vi "WAV.vi"(0 "System no.":i32=1 min=1 max=4 step=1, 2 "Waveform":u16(ring) items=["SIN", "POL", "TAN", "PNT", "SIN_P", "LIN", "RAMP", "NOISE", "SWEEP"], 3 "Affected axes":string[](array[string]), 4 "Append? (&)":bool, 5 "Add? (+)":bool, 6 "No.of digits":i16=3, 7 "error in":errorcluster, 8 "Xo":i32, 9 "N":i32=1000, 10 "Nmax for PNT":i32=5, 11 "Segment length":i32 min=0 step=1, 12 "PNT Parameters":cluster{"Ao..An-1":dbl[]}={"Ao..An-1"=[0.001, 0.002, 0.003, 0.004, 0.005, 0.006, 0.007, 0.008, 0.009, 0.01]} {"Ao..An-1" format="%.6f"}, 13 "SIN Parameters":T3={"A"=5.0, "N"=7692.0, "xo"=0.0, "Phi"=0.0, "B"=5.0} {"B" format="%.6f"; "Phi" format="%.6f"; "xo" format="%.6f"; "N" format="%.6f"; "A" format="%.6f"}, 14 "TAN Parameters":T3={"A"=10.0, "N"=6283.0, "xo"=0.0, "Phi"=0.0, "B"=0.0} {"B" format="%.6f"; "Phi" format="%.6f"; "xo" format="%.6f"; "N" format="%.6f"; "A" format="%.6f"}, 15 "POL Parameters":T2={"xo"=0.0, "Ao"=0.0, "A1"=0.01, "A2"=0.0, "A3"=0.0, "A4"=0.0, "A5"=0.0} {"A5" format="%.12f"; "A4" format="%.12f"; "A3" format="%.12f"; "A2" format="%.12f"; "A1" format="%.12f"; "Ao" format="%.12f"; "xo" format="%.12f"}, 16 "RAMP Parameters":cluster{"C":dbl, "J":dbl, "A":dbl, "O":dbl}={"C"=500.0, "J"=0.0, "A"=5.0, "O"=0.0} {"O" format="%.6f"; "A" format="%.6f"; "J" format="%.6f"; "C" format="%.6f"}, 17 "SIN_P Parameters":cluster{"C":dbl, "A":dbl, "O":dbl}={"C"=500.0, "A"=5.0, "O"=0.0} {"O" format="%.6f"; "A" format="%.6f"; "C" format="%.6f"}, 18 "LIN Parameters":cluster{"J":dbl, "A":dbl, "O":dbl}={"J"=0.0, "A"=5.0, "O"=0.0} {"O" format="%.6f"; "A" format="%.6f"; "J" format="%.6f"}, 19 "NOISE Parameters":cluster{"A":dbl, "O":dbl}={"A"=5.0, "O"=0.0} {"O" format="%.6f"; "A" format="%.6f"}, 26 "SWEEP Parameters":T1={"Start"=0, "Stop"=0, "T"=0, "A"=5.0, "O"=0.0} {"O" format="%.6f"; "A" format="%.6f"}) -> (20 "Controller error":bool, 27 "error out":errorcluster)   [LabVIEW 2020]
doc: "Defines or modifies a stored waveform for one or more axes. Please refer to the GCS DLL manual or to the user manual for a description of waveform parameters, units and restrictions. No. of digits is the number of digits after the decimal point in the parameter value(s) that will be sent. Controller error is TRUE if selected system reports error code not equal to 0.\nC-413: Affected axis is identical with wave table number. 8 waves can be defined in total. Use WSL.vi to connect wave table to wave generator. See User Manual for details.\nWaveform can be: SIN _P , RAMP, LIN or PNT. \nC-886: Affected axis is identical with wave table number. 100 waves can bedefined in total. Use WSL.vi to connect wave table to wave generator.\nWaveform can be: SIN_P, PNT, LIN, or RAMP. Check MAN? WAV answer to find out which waveforms are supported.\nC-887: Affected axis is identical with wave table number. 100 waves can bedefined in total. Use WSL.vi to connect wave table to wave generator.\nWaveform can be: SIN_P, PNT, LIN, or RAMP. Check MAN? WAV answer to find out which waveforms are supported.. \nC-891: Affected axis is identical with wave table number. 40 waves can be defined in total. Use WSL.vi to connect wave table to wave generator.Waveform can be: SIN_P, RAMP, or LIN. \n\nE-516: Waveform can be: SIN, TAN, POL or PNT.\nThe following parameters are equivalent (see GCS DLL manual):\nAffected axes = szAxes, Xo = nStart, N = nLength, Add? = Add, \nPNT Parameters = pPoints (PNT parameters is an array consisting of single data points which will be sent in groups of Nmax for PNT data points.)\nE-517, E-518: Affected axis is identical with wave table number, which can be 1 to 3. One wave table number per command call allowed only.\nWaveform can be: SIN_P, RAMP or LIN. For SIN, TAN, POL and PNT Segment length must be zero.\nE-709: Affected axis is identical with wave table number. 6 waves can be defined in total. Use WSL.vi to connect wave table to wave generator. Waveforms are automatically stored in non-volatile memory. Note that the number of write cycles is limited. See user manual for details.\nWaveform can be: SIN_P, RAMP, or LIN. \n\nE-710: Affected axis is identical with wave table number.\nWaveform can be: SIN_P, RAMP, LIN or PNT. \nThe length of the wave to define must be less than the value defined with WMS.vi.\n\nE-712: Affected axis is identical with wave table number. 90 waves can be defined in total. Use WSL.vi to connect wave table to wave generator.\nWaveform can be: SIN_P, RAMP, LIN, NOISE or PNT. \nE-725: Affected axis is identical with wave table number. 30 waves can be defined in total. Use WSL.vi to connect wave table to wave generator.\nWaveform can be: SIN_P, RAMP, LIN, NOISE or PNT. \nE-727: Affected axis is identical with wave table number. 40 waves can be defined in total. Use WSL.vi to connect wave table to wave generator.\nWaveform can be: SIN_P, RAMP, LIN, NOISE or PNT. \nE-753: Affected axis is identical with wave table number. 10 waves can be defined in total. Use WSL.vi to connect wave table to wave generator.\nWaveform can be: SIN_P, RAMP, LIN, NOISE or PNT. \nE-754: Affected axis is identical with wave table number. 10 waves can be defined in total. Use WSL.vi to connect wave table to wave generator.\nWaveform can be: SIN_P, PNT, RAMP, LIN, NOISE or SWEEP. \nValid for SWEEP: Affected axes, Append?, SWEEP Parameters. See controller user manual for details.\n\nE-761: Affected axis is identical with wave table number.\nWaveform can be: SIN_P, RAMP, LIN, PNT or POL. \nGeneral: The following parameters are equivalent (see GCS DLL manual): \nAffected axes = szWaveTableIds, Xo = iOffsetOfFirstPointInWaveTable, N = iNumberOfPoints, Append? = iAddAppendWave, C = iCenterPointOfWave, J = iNumberOfSpeedUpDownPointsInWave, A = dAmplitudeOfWave, O = dOffsetOfWave (is only valid if a wave segment is being concatenated to an existing wave, i.e. Append? = TRUE), Segment length = iSegmentLength, PNT Parameters = pdWavePoints (PNT parameters is an array consisting of single data points which will be sent in groups of Nmax for PNT data points.)\nValid for SIN: Affected axes, No. of digits, Xo, N, Add?, SIN Parameters (A, N, Xo, Phi and B)\nValid for LIN: Affected axes, No. of digits, Xo, N, Append?, Segment length, LIN Parameters (J, A and O)\nValid for TAN: Affected axes, No. of digits, Xo, N, Add?, TAN Parameters (A, N, Xo, Phi and B)\nValid for PNT: see above."
uses:
  Controller names.ctl
  Global2 (Array).vi
panel:
  # "This vi defines or modifies a stored waveform for one or more axes. Please refer to the system manual for a description of waveform parameters, \nunits and restrictions."
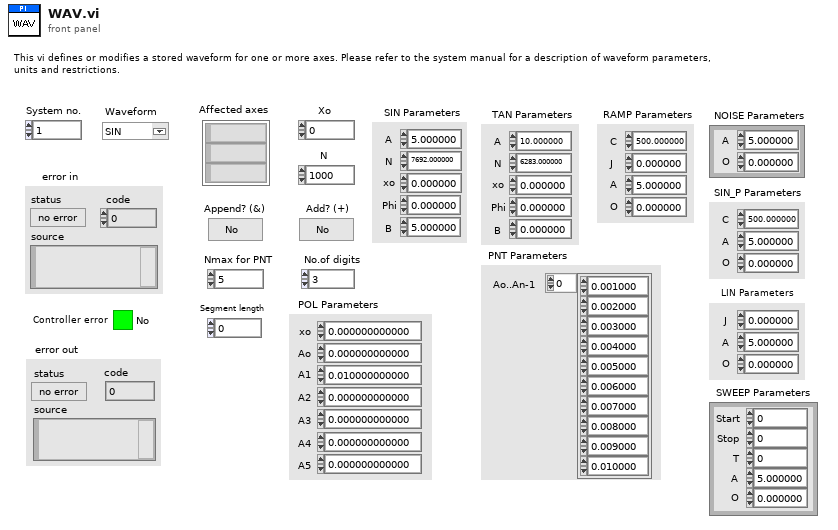
[diagram p1: front panel]
types:
  T1 = cluster{"Start":i32, "Stop":i32, "T":i32, "A":dbl, "O":dbl}
  T2 = cluster{"xo":dbl, "Ao":dbl, "A1":dbl, "A2":dbl, "A3":dbl, "A4":dbl, "A5":dbl}
  T3 = cluster{"A":dbl, "N":dbl, "xo":dbl, "Phi":dbl, "B":dbl}
  T4 = typedef "Controller names.ctl" = enum16{"None", "Analog", "C-702", "C-413", "C-414", "C-843", "C-843.PM", "C-844", "C-848", "C-865", "C-866", "C-867", "C-877", "C-880", "C-884", "C-885", "C-886", "C-887", "C-891", "E-135", "E-516", "E-517", "E-518", "E-709", "E-710", "E-712", "E-725", "E-727", "E-753", "E-754", "E-755", "E-761", "E-816", "E-861", "E-870", "E-871", "E-872", "E-873", "E-874", "F-206", "HydraPollux", "M-840", "M-850", "M-8X0", "Mercury", "Mercury_GCS", "PI_GCS2"}
  T5 = enum16{"Disable error check", "Force error check", "Use global settings"}
  T6 = cluster{"Conn. axes":string[], "Controller name":T4}[]
  T7 = cluster{"Conn. axes":string[], "Controller name":T4}
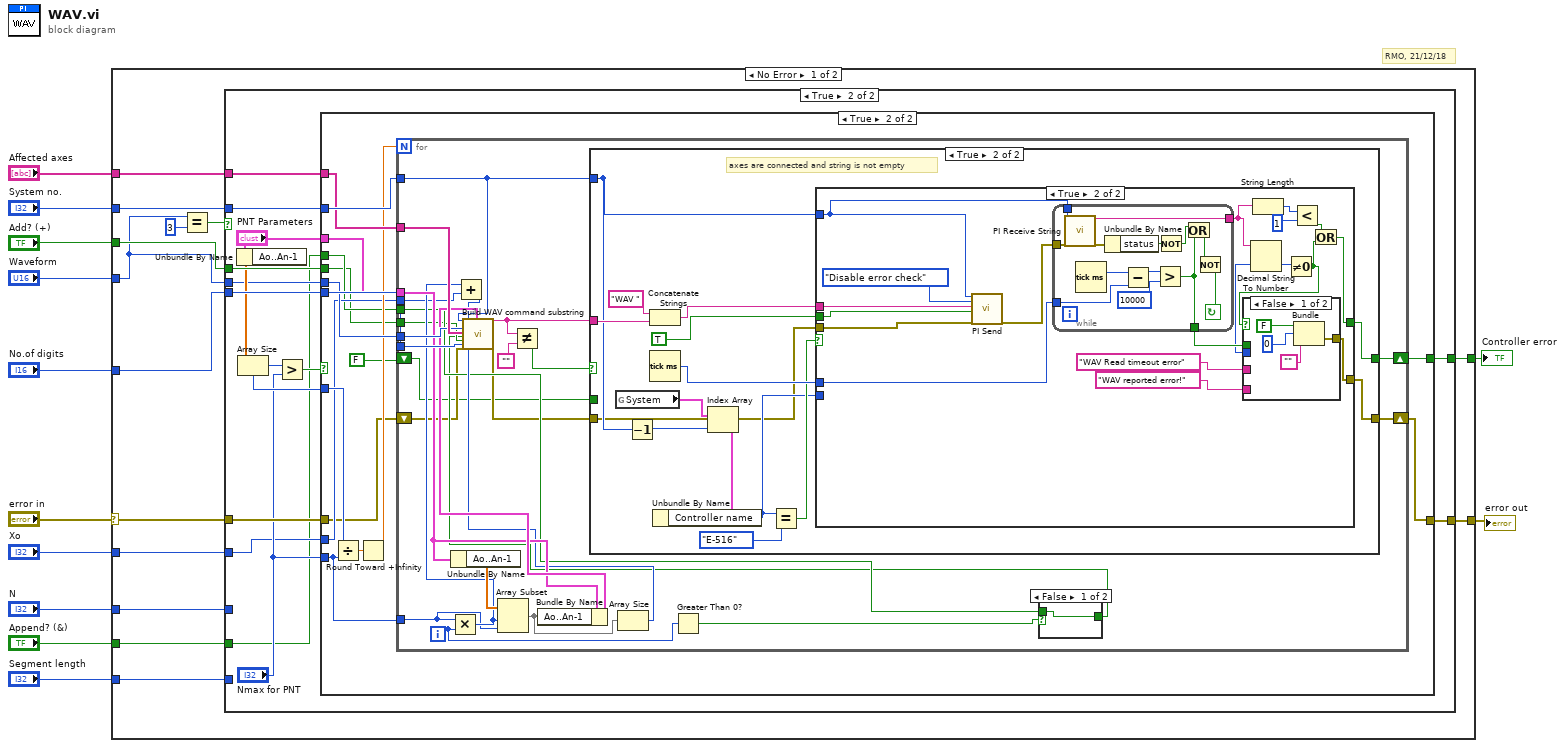
[diagram p0: block diagram]
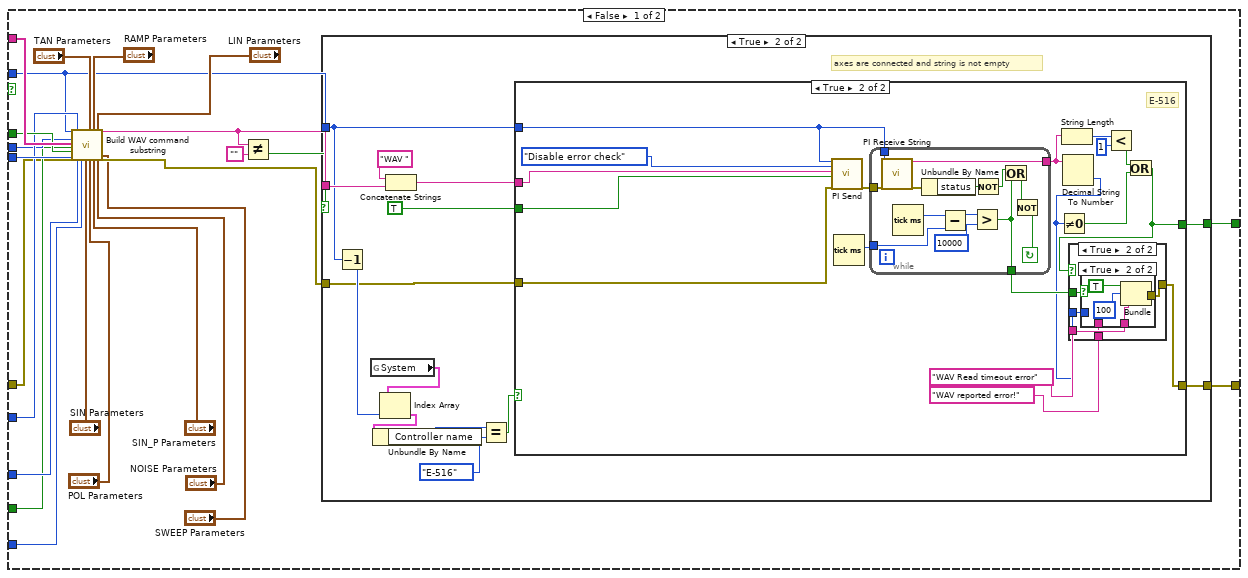
[diagram p2: hidden frame]
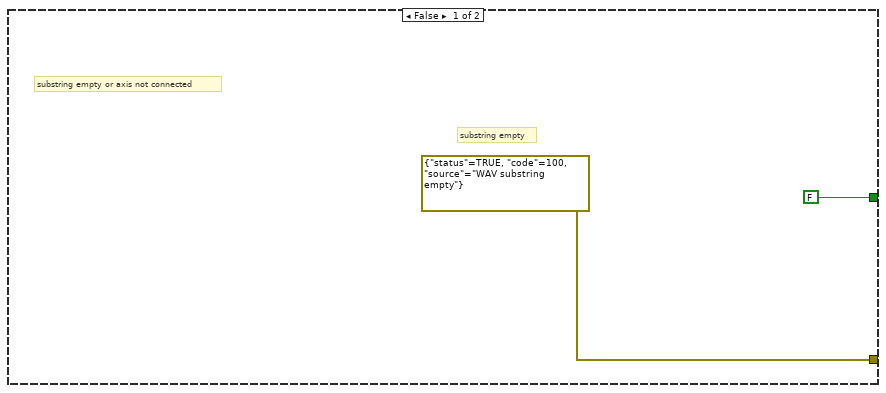
[diagram p3: hidden frame]
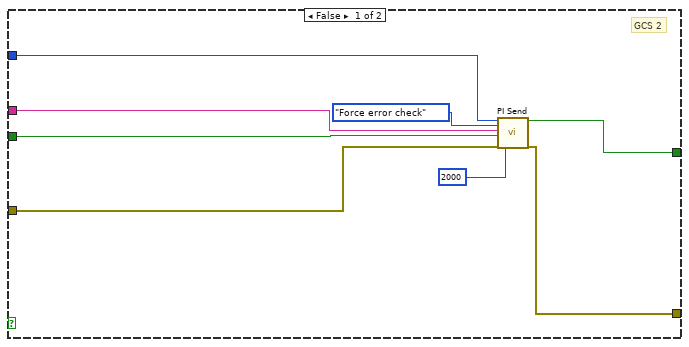
[diagram p4: hidden frame]
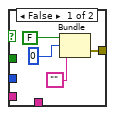
[diagram p5: hidden frame]
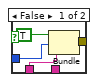
[diagram p6: hidden frame]
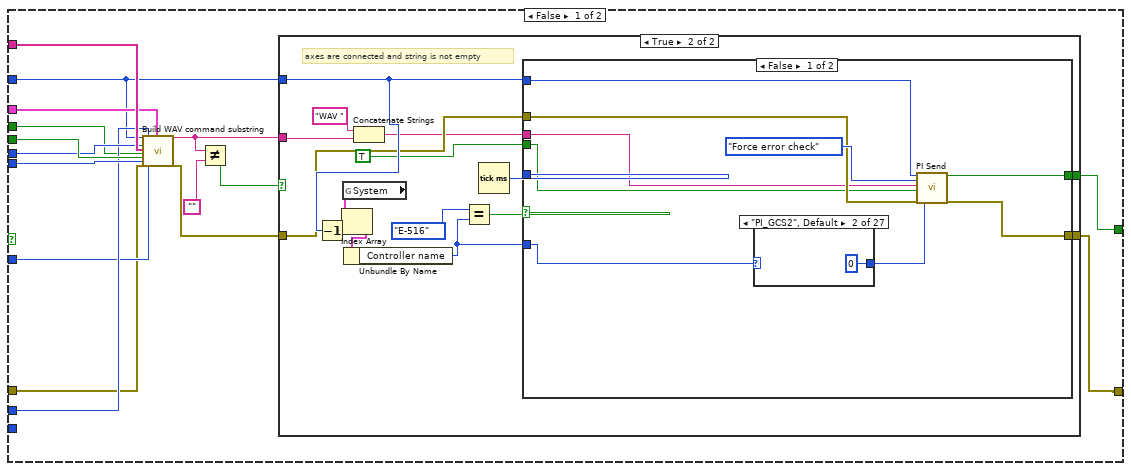
[diagram p7: hidden frame]
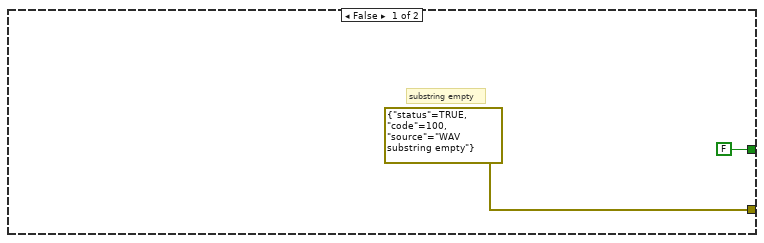
[diagram p8: hidden frame]
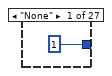
[diagram p9: hidden frame]
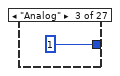
[diagram p10: hidden frame]
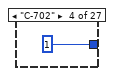
[diagram p11: hidden frame]
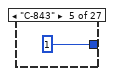
[diagram p12: hidden frame]
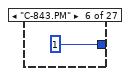
[diagram p13: hidden frame]
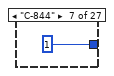
[diagram p14: hidden frame]
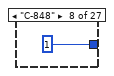
[diagram p15: hidden frame]
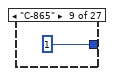
[diagram p16: hidden frame]
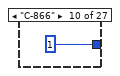
[diagram p17: hidden frame]
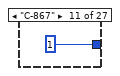
[diagram p18: hidden frame]
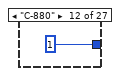
[diagram p19: hidden frame]
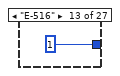
[diagram p20: hidden frame]
diagram:
  # "RMO, 21/12/18"
  n1 = case shown="No Error" "error in" {
    selector: "error in" -> [w13 w406]
    tunnel: [w26 w406] -> w2
    tunnel: "System no." -> [w25 _]
    tunnel: "Affected axes" -> [w24 _]
    tunnel: "Add? (+)" -> [w23 _]
    tunnel: "No.of digits" -> [w22 _]
    tunnel: "Xo" -> [w21 _]
    tunnel: "N" -> [w20 _]
    tunnel: "Waveform" -> [w19 _]
    tunnel: [w16 FALSE] -> w6
    tunnel: "Append? (&)" -> [w15 _]
    tunnel: "Segment length" -> [w14 _]
    frame No Error {
      n2 = Equal?(x=w19, y=u16 3) -> (x = y?=w17:bool)
      n3 = case shown="True" w17 {
        tunnel: [w50 w137] -> w26
        tunnel: w13 -> [w29 w136]
        tunnel: w25 -> [w31 w135]
        tunnel: w24 -> [w47 w134]
        tunnel: w23 -> [w46 w133]
        tunnel: w22 -> [w45 w132]
        tunnel: w21 -> [w44 w124]
        tunnel: w20 -> [w42 _]
        tunnel: w19 -> [w39 w130]
        tunnel: [w38 w125] -> w16
        tunnel: w15 -> [w37 w123]
        tunnel: w14 -> [w33 _]
        frame False {
          n4 = call "Build WAV command substring.vi"("System no."=w31, "Waveform"=w39, "Axes to set"=w47, "Append? (&)"=w37, "Add? (+)"=w46, "No. of digits"=w45, "error in (no error)"=w29, "Xo"=w44, "N"=w42, "Segment length"=w33, "SIN Parameters"="SIN Parameters", "TAN Parameters"="TAN Parameters", "POL Parameters"="POL Parameters", "RAMP Parameters"="RAMP Parameters", "SIN_P Parameters"="SIN_P Parameters", "LIN Parameters"="LIN Parameters", "NOISE Parameters"="NOISE Parameters", "SWEEP Parameters"="SWEEP Parameters") -> ("WAV command substring"=w48:string, "error out"=w28:errorcluster)  [unwired: 1 in, 7 out]
          n5 = Not Equal?(x=w48, y="") -> (x != y?=w32:bool)
          n6 = case shown="True" w32 {
            tunnel: w48 -> [_ w65]
            tunnel: [errorcluster {"status"=TRUE, "code"=100, "source"="WAV substring empty"} ("error out") w64] -> w50
            tunnel: w28 -> [_ w55]
            tunnel: w31 -> [_ w60]
            tunnel: [FALSE w63] -> w38
            frame False {
              # "substring empty"
              # "substring empty or axis not connected"
            }
            frame True {
              # "axes are connected and string is not empty"
              n7 = Decrement(x=w60) -> (x-1=w56:i32)
              n8 = global read "Global2 (Array).vi" "System"() -> (w59:T6)
              n9 = Index Array(array=w59, index=w56) -> (element=w58:T7)
              n10 = Unbundle By Name(w58) -> ("Controller name"=w57:T4)
              n11 = Concatenate Strings("WAV ", w65) -> (w54:string)
              n12 = Equal?(x=w57, y=Controller_names."E-516" ("System 1")) -> (x = y?=w61:bool)
              n13 = case shown="True" w61 {
                tunnel: w55 -> [w74 w79]
                tunnel: [w68 w87] -> w64
                tunnel: [w69 w81] -> w63
                tunnel: w60 -> [w73 w76]
                tunnel: w54 -> [w72 w77]
                tunnel: TRUE ("Attach Linefeed?") -> [w71 w78]
                frame False {
                  # "GCS 2"
                  n14 = call "PI Send.vi"("System no."=w73, "Error check settings"=T5."Force error check", "String to send"=w72, "Attach termination char.?"=w71, "error in"=w74, "Delay before error check (ms)"=u32 2000 ("milliseconds to wait")) -> ("Controller error"=w69:bool, "error out"=w68:errorcluster)  [unwired: 12 out]
                }
                frame True {
                  # "E-516"
                  n15 = call "PI Send.vi"("System no."=w76, "Error check settings"=T5."Disable error check", "String to send"=w77, "Attach termination char.?"=w78, "error in"=w79) -> ("error out"=w80:errorcluster)  [unwired: 1 in, 13 out]
                  n16 = Tick Count (ms)() -> (millisecond timer value=w92:u32)
                  n17 = while {
                    tunnel: [w93] -> w91
                    tunnel: [w94] -> w86
                    tunnel: w76 -> [w95]
                    tunnel: w80 -> [w96]
                    tunnel: w92 -> [w97]
                    stop <- w98 continue-if-true
                    n18 = call "PI Receive String.vi"("System no."=w95, "error in"=w96) -> ("String read"=w94:string, "error out"=w105:errorcluster)  [unwired: 1 in, 15 out]
                    n19 = Tick Count (ms)() -> (millisecond timer value=w103:u32)
                    n20 = Unbundle By Name(w105) -> ("status"=w104:bool)
                    n21 = Subtract(x=w103, y=w97) -> (x-y=w102:u32)
                    n22 = Greater?(x=w102, y=u32 10000) -> (0:w93:bool)
                    n23 = Not(x=w104) -> (.not. x?=w100:bool)
                    n24 = Or(x=w100, y=w93) -> (x .or. y?=w99:bool)
                    n25 = Not(x=w99) -> (.not. x?=w98:bool)
                  }
                  n26 = String Length(string=w86) -> (length=w85:i32)
                  n27 = Decimal String To Number(string=w86) -> (number=w89:i32)  [unwired: 3 out]
                  n28 = Not Equal To 0?(x=w89) -> (x != 0?=w82:bool)
                  n29 = Less?(x=w85, y=1) -> (x < y?=w83:bool)
                  n30 = Or(x=w83, y=w82) -> (x .or. y?=w81:bool)
                  n31 = case shown="True" w81 {
                    tunnel: w91 -> [_ w114]
                    tunnel: "WAV Read timeout error" -> [_ w113]
                    tunnel: w89 -> [_ w112]
                    tunnel: "WAV reported error!" -> [_ w111]
                    tunnel: [w106 w110] -> w87
                    frame False {
                      n32 = Bundle(FALSE, 0, "") -> (w106:errorcluster)  [unwired: 1 out]
                    }
                    frame True {
                      n33 = case shown="True" w114 {
                        tunnel: w113 -> [_ w120]
                        tunnel: w112 -> [w117 _]
                        tunnel: w111 -> [w116 _]
                        tunnel: [w115 w119] -> w110
                        frame False {
                          n34 = Bundle(TRUE, w117, w116) -> (w115:errorcluster)  [unwired: 1 out]
                        }
                        frame True {
                          n35 = Bundle(TRUE, 100, w120) -> (w119:errorcluster)  [unwired: 1 out]
                        }
                      }
                    }
                  }
                }
              }
            }
          }
        }
        frame True {
          n36 = Unbundle By Name("PNT Parameters") -> ("Ao..An-1"=w131:dbl[])
          n37 = Array Size(array=w131) -> (size(s)=w127:i32)
          n38 = Greater?(x=w127, y="Nmax for PNT") -> (0:w128:bool)
          n39 = case shown="True" w128 {
            tunnel: [w153 w258] -> w137
            tunnel: w136 -> [w139 w259]
            tunnel: w135 -> [w140 w270]
            tunnel: w134 -> [w150 w269]
            tunnel: w133 -> [w149 w256]
            tunnel: w132 -> [w148 w268]
            tunnel: w130 -> [w147 w267]
            tunnel: "PNT Parameters" -> [w146 w266]
            tunnel: w127 -> [w143 w265]
            tunnel: "Nmax for PNT" -> [_ w262]
            tunnel: [w145 w261] -> w125
            tunnel: w124 -> [w144 w260]
            tunnel: w123 -> [w142 w257]
            frame False {
              n40 = call "Build WAV command substring.vi"("System no."=w140, "Waveform"=w147, "Axes to set"=w150, "Append? (&)"=w142, "Add? (+)"=w149, "No. of digits"=w148, "error in (no error)"=w139, "Xo"=w144, "N"=w143, "PNT Parameters"=w146) -> ("WAV command substring"=w151:string, "error out"=w138:errorcluster)  [unwired: 9 in, 7 out]
              n41 = Not Equal?(x=w151, y="") -> (x != y?=w141:bool)
              n42 = case shown="True" w141 {
                tunnel: w151 -> [_ w169]
                tunnel: [errorcluster {"status"=TRUE, "code"=100, "source"="WAV substring empty"} ("error out") w159] -> w153
                tunnel: w138 -> [_ w158]
                tunnel: w140 -> [_ w162]
                tunnel: [FALSE w160] -> w145
                frame False {
                  # "substring empty"
                }
                frame True {
                  # "axes are connected and string is not empty"
                  n43 = Decrement(x=w162) -> (x-1=w165:i32)
                  n44 = global read "Global2 (Array).vi" "System"() -> (w167:T6)
                  n45 = Index Array(array=w167, index=w165) -> (element=w166:T7)
                  n46 = Unbundle By Name(w166) -> ("Controller name"=w161:T4)
                  n47 = Concatenate Strings("WAV ", w169) -> (w157:string)
                  n48 = Equal?(x=Controller_names."E-516" ("System 1"), y=w161) -> (x = y?=w163:bool)
                  n49 = Tick Count (ms)() -> (millisecond timer value=w164:u32)
                  n50 = case shown="False" w163 {
                    tunnel: w164 -> [_ w224]
                    tunnel: w158 -> [w177 w212]
                    tunnel: w162 -> [w174 w210]
                    tunnel: w161 -> [w171 _]
                    tunnel: [w172 w219] -> w160
                    tunnel: [w173 w218] -> w159
                    tunnel: w157 -> [w176 w208]
                    tunnel: TRUE ("Attach Linefeed?") -> [w175 w207]
                    frame False {
                      n51 = case shown="\"PI_GCS2\", Default" w171 {
                        tunnel: [u32 1 ("milliseconds to wait") u32 0 ("milliseconds to wait") u32 1 ("milliseconds to wait") u32 1 ("milliseconds to wait") u32 1 ("milliseconds to wait") u32 1 ("milliseconds to wait") u32 1 ("milliseconds to wait") u32 1 ("milliseconds to wait") u32 1 ("milliseconds to wait") u32 1 ("milliseconds to wait") u32 1 ("milliseconds to wait") u32 1 ("milliseconds to wait") u32 1 ("milliseconds to wait") u32 1 ("milliseconds to wait") u32 2000 ("milliseconds to wait") u32 1 ("milliseconds to wait") u32 1 ("milliseconds to wait") u32 2000 ("milliseconds to wait") u32 2000 ("milliseconds to wait") u32 1 ("milliseconds to wait") u32 2000 ("milliseconds to wait") u32 2000 ("milliseconds to wait") u32 1 ("milliseconds to wait") u32 1 ("milliseconds to wait") u32 1 ("milliseconds to wait") u32 1 ("milliseconds to wait") u32 1 ("milliseconds to wait")] -> w178
                        frame "None" {
                        }
                        frame "PI_GCS2", Default {
                        }
                        frame "Analog" {
                        }
                        frame "C-702" {
                        }
                        frame "C-843" {
                        }
                        frame "C-843.PM" {
                        }
                        frame "C-844" {
                        }
                        frame "C-848" {
                        }
                        frame "C-865" {
                        }
                        frame "C-866" {
                        }
                        frame "C-867" {
                        }
                        frame "C-880" {
                        }
                        frame "E-516" {
                        }
                        frame "E-517" {
                        }
                        frame "E-710" {
                        }
                        frame "E-712" {
                        }
                        frame "E-725" {
                        }
                        frame "E-753" {
                        }
                        frame "E-755" {
                        }
                        frame "E-761" {
                        }
                        frame "E-816" {
                        }
                        frame "E-861" {
                        }
                        frame "F-206" {
                        }
                        frame "M-840" {
                        }
                        frame "M-850" {
                        }
                        frame "M-8X0" {
                        }
                        frame "Mercury" {
                        }
                      }
                      n52 = call "PI Send.vi"("System no."=w174, "Error check settings"=T5."Force error check", "String to send"=w176, "Attach termination char.?"=w175, "error in"=w177, "Delay before error check (ms)"=w178) -> ("Controller error"=w172:bool, "error out"=w173:errorcluster)  [unwired: 12 out]
                    }
                    frame True {
                      n53 = call "PI Send.vi"("System no."=w210, "Error check settings"=T5."Disable error check", "String to send"=w208, "Attach termination char.?"=w207, "error in"=w212) -> ("error out"=w211:errorcluster)  [unwired: 1 in, 13 out]
                      n54 = while {
                        tunnel: [w242] -> w216
                        tunnel: [w243] -> w220
                        tunnel: w210 -> [w244]
                        tunnel: w211 -> [w245]
                        tunnel: w224 -> [w246]
                        stop <- w247 continue-if-true
                        n55 = call "PI Receive String.vi"("System no."=w244, "error in"=w245) -> ("String read"=w243:string, "error out"=w254:errorcluster)  [unwired: 1 in, 15 out]
                        n56 = Tick Count (ms)() -> (millisecond timer value=w252:u32)
                        n57 = Unbundle By Name(w254) -> ("status"=w253:bool)
                        n58 = Subtract(x=w252, y=w246) -> (x-y=w251:u32)
                        n59 = Greater?(x=w251, y=u32 10000) -> (0:w242:bool)
                        n60 = Not(x=w253) -> (.not. x?=w249:bool)
                        n61 = Or(x=w249, y=w242) -> (x .or. y?=w248:bool)
                        n62 = Not(x=w248) -> (.not. x?=w247:bool)
                      }
                      n63 = Decimal String To Number(string=w220) -> (number=w213:i32)  [unwired: 3 out]
                      n64 = String Length(string=w220) -> (length=w223:i32)
                      n65 = Not Equal To 0?(x=w213) -> (x != 0?=w217:bool)
                      n66 = case shown="False" w217 {
                        tunnel: [w225 w233] -> w218
                        tunnel: w216 -> [_ w232]
                        tunnel: "WAV Read timeout error" -> [_ w231]
                        tunnel: "WAV reported error!" -> [_ w230]
                        tunnel: w213 -> [_ w229]
                        frame False {
                          n67 = Bundle(FALSE, 0, "") -> (w225:errorcluster)  [unwired: 1 out]
                        }
                        frame True {
                          n68 = case shown="True" w232 {
                            tunnel: [w234 w238] -> w233
                            tunnel: w231 -> [_ w239]
                            tunnel: w230 -> [w236 _]
                            tunnel: w229 -> [w235 _]
                            frame False {
                              n69 = Bundle(TRUE, w235, w236) -> (w234:errorcluster)  [unwired: 1 out]
                            }
                            frame True {
                              n70 = Bundle(TRUE, 100, w239) -> (w238:errorcluster)  [unwired: 1 out]
                            }
                          }
                        }
                      }
                      n71 = Less?(x=w223, y=1) -> (x < y?=w221:bool)
                      n72 = Or(x=w221, y=w217) -> (x .or. y?=w219:bool)
                    }
                  }
                }
              }
            }
            frame True {
              n73 = Divide(x=w265, y=w262) -> (x/y=w264:dbl)
              n74 = Round Toward +Infinity(x=w264) -> (ceil(x): smallest int >= x=w263:dbl)
              n75 = for {
                N: w263 -> [_]
                tunnel: w270 -> [w279]
                tunnel: w269 -> [w294]
                tunnel: w256 -> [w275]
                tunnel: w268 -> [w293]
                tunnel: w267 -> [w292]
                tunnel: w266 -> [w289]
                tunnel: w262 -> [w283]
                tunnel: w260 -> [w286]
                shift-right: [w281] -> w258
                shift-left: w259 -> [w273]
                tunnel: w257 -> [w276]
                shift-right: [w288] -> w261
                shift-left: FALSE -> [w271]
                i -> [w278]
                n76 = Multiply(x=w283, y=w278) -> (x*y=w287:i32)
                n77 = Unbundle By Name(w289) -> ("Ao..An-1"=w291:dbl[])
                n78 = Add(x=w287, y=w286) -> (x+y=w285:i32)
                n79 = Array Subset(array=w291, index=w287, length=w283) -> (w284:dbl[])
                n80 = Bundle By Name(cluster=w289, "Ao..An-1"=w284) -> (w290:cluster{"Ao..An-1":dbl[]})
                n81 = Array Size(array=w284) -> (size(s)=w282:i32)
                n82 = Greater Than 0?(x=w278) -> (x > 0?=w277:bool)
                n83 = case shown="False" w277 {
                  tunnel: w276 -> [w297 _]
                  tunnel: [w297 TRUE ("Add? (+)")] -> w274
                  frame False {
                  }
                  frame True {
                  }
                }
                n84 = call "Build WAV command substring.vi"("System no."=w279, "Waveform"=w292, "Axes to set"=w294, "Append? (&)"=w274, "Add? (+)"=w275, "No. of digits"=w293, "error in (no error)"=w273, "Xo"=w285, "N"=w282, "PNT Parameters"=w290) -> ("WAV command substring"=w295:string, "error out"=w272:errorcluster)  [unwired: 9 in, 7 out]
                n85 = Not Equal?(x=w295, y="") -> (x != y?=w280:bool)
                n86 = case shown="True" w280 {
                  tunnel: w295 -> [_ w320]
                  tunnel: [w302 w310] -> w281
                  tunnel: w272 -> [w300 w309]
                  tunnel: w279 -> [_ w315]
                  tunnel: [w301 w311] -> w288
                  tunnel: w271 -> [w299 _]
                  frame False {
                    n87 = case shown="False" w299 {
                      selector: w299 -> [w303 w306]
                      tunnel: [errorcluster {"status"=TRUE, "code"=100, "source"="WAV substring empty"} ("error out") w305] -> w302
                      tunnel: [w303 w306] -> w301
                      tunnel: w300 -> [_ w305]
                      frame False {
                        # "substring empty"
                      }
                      frame True {
                      }
                    }
                  }
                  frame True {
                    # "axes are connected and string is not empty"
                    n88 = global read "Global2 (Array).vi" "System"() -> (w316:T6)
                    n89 = Decrement(x=w315) -> (x-1=w314:i32)
                    n90 = Concatenate Strings("WAV ", w320) -> (w308:string)
                    n91 = Tick Count (ms)() -> (millisecond timer value=w319:u32)
                    n92 = Index Array(array=w316, index=w314) -> (element=w313:T7)
                    n93 = Unbundle By Name(w313) -> ("Controller name"=w312:T4)
                    n94 = Equal?(x=w312, y=Controller_names."E-516" ("System 1")) -> (x = y?=w317:bool)
                    n95 = case shown="True" w317 {
                      tunnel: w319 -> [_ w375]
                      tunnel: w309 -> [w329 w363]
                      tunnel: w315 -> [w330 w360]
                      tunnel: w312 -> [w328 _]
                      tunnel: [w326 w370] -> w311
                      tunnel: [w327 w369] -> w310
                      tunnel: w308 -> [w324 w361]
                      tunnel: TRUE ("Attach Linefeed?") -> [w323 w358]
                      frame False {
                        n96 = case shown="\"C-843\"" w328 {
                          tunnel: [u32 1 ("milliseconds to wait") u32 0 ("milliseconds to wait") u32 1 ("milliseconds to wait") u32 1 ("milliseconds to wait") u32 1 ("milliseconds to wait") u32 1 ("milliseconds to wait") u32 1 ("milliseconds to wait") u32 1 ("milliseconds to wait") u32 1 ("milliseconds to wait") u32 1 ("milliseconds to wait") u32 1 ("milliseconds to wait") u32 1 ("milliseconds to wait") u32 1 ("milliseconds to wait") u32 1 ("milliseconds to wait") u32 2000 ("milliseconds to wait") u32 1 ("milliseconds to wait") u32 1 ("milliseconds to wait") u32 2000 ("milliseconds to wait") u32 2000 ("milliseconds to wait") u32 1 ("milliseconds to wait") u32 2000 ("milliseconds to wait") u32 2000 ("milliseconds to wait") u32 1 ("milliseconds to wait") u32 1 ("milliseconds to wait") u32 1 ("milliseconds to wait") u32 1 ("milliseconds to wait") u32 1 ("milliseconds to wait")] -> w322
                          frame "None" {
                          }
                          frame "PI_GCS2", Default {
                          }
                          frame "Analog" {
                          }
                          frame "C-702" {
                          }
                          frame "C-843" {
                          }
                          frame "C-843.PM" {
                          }
                          frame "C-844" {
                          }
                          frame "C-848" {
                          }
                          frame "C-865" {
                          }
                          frame "C-866" {
                          }
                          frame "C-867" {
                          }
                          frame "C-880" {
                          }
                          frame "E-516" {
                          }
                          frame "E-517" {
                          }
                          frame "E-710" {
                          }
                          frame "E-712" {
                          }
                          frame "E-725" {
                          }
                          frame "E-753" {
                          }
                          frame "E-755" {
                          }
                          frame "E-761" {
                          }
                          frame "E-816" {
                          }
                          frame "E-861" {
                          }
                          frame "F-206" {
                          }
                          frame "M-840" {
                          }
                          frame "M-850" {
                          }
                          frame "M-8X0" {
                          }
                          frame "Mercury" {
                          }
                        }
                        n97 = call "PI Send.vi"("System no."=w330, "Error check settings"=T5."Force error check", "String to send"=w324, "Attach termination char.?"=w323, "error in"=w329, "Delay before error check (ms)"=w322) -> ("Controller error"=w326:bool, "error out"=w327:errorcluster)  [unwired: 12 out]
                      }
                      frame True {
                        n98 = call "PI Send.vi"("System no."=w360, "Error check settings"=T5."Disable error check", "String to send"=w361, "Attach termination char.?"=w358, "error in"=w363) -> ("error out"=w362:errorcluster)  [unwired: 1 in, 13 out]
                        n99 = while {
                          tunnel: [w393] -> w367
                          tunnel: [w394] -> w371
                          tunnel: w360 -> [w395]
                          tunnel: w362 -> [w396]
                          tunnel: w375 -> [w397]
                          stop <- w398 continue-if-true
                          n100 = call "PI Receive String.vi"("System no."=w395, "error in"=w396) -> ("String read"=w394:string, "error out"=w405:errorcluster)  [unwired: 1 in, 15 out]
                          n101 = Tick Count (ms)() -> (millisecond timer value=w403:u32)
                          n102 = Unbundle By Name(w405) -> ("status"=w404:bool)
                          n103 = Subtract(x=w403, y=w397) -> (x-y=w402:u32)
                          n104 = Greater?(x=w402, y=u32 10000) -> (0:w393:bool)
                          n105 = Not(x=w404) -> (.not. x?=w400:bool)
                          n106 = Or(x=w400, y=w393) -> (x .or. y?=w399:bool)
                          n107 = Not(x=w399) -> (.not. x?=w398:bool)
                        }
                        n108 = Decimal String To Number(string=w371) -> (number=w364:i32)  [unwired: 3 out]
                        n109 = String Length(string=w371) -> (length=w374:i32)
                        n110 = Not Equal To 0?(x=w364) -> (x != 0?=w368:bool)
                        n111 = case shown="False" w368 {
                          tunnel: [w376 w384] -> w369
                          tunnel: w367 -> [_ w383]
                          tunnel: "WAV Read timeout error" -> [_ w382]
                          tunnel: "WAV reported error!" -> [_ w381]
                          tunnel: w364 -> [_ w380]
                          frame False {
                            n112 = Bundle(FALSE, 0, "") -> (w376:errorcluster)  [unwired: 1 out]
                          }
                          frame True {
                            n113 = case shown="False" w383 {
                              tunnel: [w385 w389] -> w384
                              tunnel: w382 -> [_ w390]
                              tunnel: w381 -> [w387 _]
                              tunnel: w380 -> [w386 _]
                              frame False {
                                n114 = Bundle(TRUE, w386, w387) -> (w385:errorcluster)  [unwired: 1 out]
                              }
                              frame True {
                                n115 = Bundle(TRUE, 100, w390) -> (w389:errorcluster)  [unwired: 1 out]
                              }
                            }
                          }
                        }
                        n116 = Less?(x=w374, y=1) -> (x < y?=w372:bool)
                        n117 = Or(x=w372, y=w368) -> (x .or. y?=w370:bool)
                      }
                    }
                  }
                }
              }
            }
          }
        }
      }
    }
    frame Error {
    }
  }
  "error out" <- w2
  "Controller error" <- w6
